vi "Plugin Configuration.UDP.Init.vi"(8 "error in (no error)":errorcluster, 10 "Port":string, 11 "IP Address":string) -> (0 "error out":errorcluster, 3 "UDP Plugin Configuration":refnum<class "Plugin Configuration.UDP.lvclass">)   [LabVIEW 2016, in "Plugin Configuration.UDP.lvclass"]
uses:
  Plugin Configuration.UDP.lvclass
  C:/Users/Ryan/Documents/Git/Sourcetree/VeriStand-Data-Sharing-Framework/Source/Classes/Plugin Model/Plugin Configuration.lvclass
  Plugin Model/Typedefs/Plugin Configuration.Typedef.URL Configuration.ctl
  Plugin Model/Plugin Configuration.lvclass/Plugin Configuration.ctl
  Plugin Model/Properties/Set URL Config.vi
  Plugin Model/Plugin Configuration.lvclass
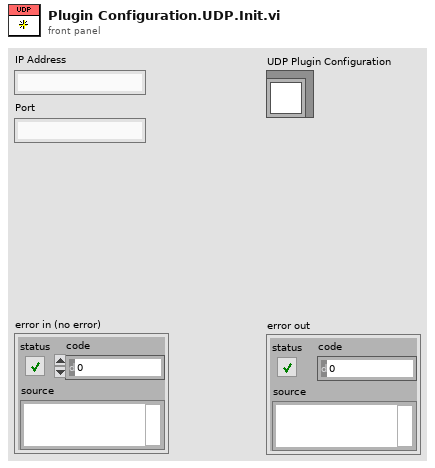
[diagram p1: front panel]
types:
  T1 = typedef "Data Sharing Framework.Configuration.lvlib/Plugin Configuration.lvclass/Plugin Configuration.Typedef.URL Configuration.ctl" = cluster{"protocol":string, "body":string}
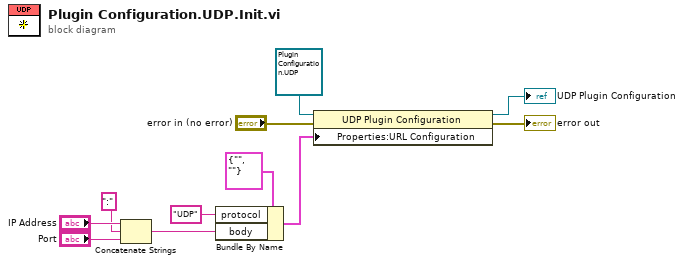
[diagram p0: block diagram]
diagram:
  n1 = Concatenate Strings("IP Address", ":", "Port") -> (w1:string)
  n2 = Bundle By Name(cluster=T1 {"protocol"="", "body"=""} ("resource name config"), "protocol"="UDP" ("resource prefix"), "body"=w1) -> (w9:T1)
  n3 = property class="UDP Plugin Configuration"(reference=refnum<class "Plugin Configuration.UDP.lvclass"> refnum ("UDP Plugin Model"), error in="error in (no error)", "Properties:URL Configuration"=w9) -> (reference out=→"UDP Plugin Configuration":refnum<class "Plugin Configuration.UDP.lvclass">, error out=→"error out":errorcluster)
